vi "List_Files.vi"(8 "error in (no error)":errorcluster, 11 "IB_Source_File in":refnum<class "IB_Source_File.lvclass">) -> (0 "error out":errorcluster, 3 "Files":T1[](array[typedef]))   [LabVIEW 2020, in "IB_Source_File.lvclass"]
uses:
  <vilib>/AppBuilder/IB_Classes/Source/File/IB_Source_File.lvclass
  <vilib>/AppBuilder/IB_Classes/Source/File/IB_Source_File.lvclass/IB_Source_File.ctl
  <resource>/Framework/Providers/Builds/Installer/CDK_sTypeDef_FileList.ctl
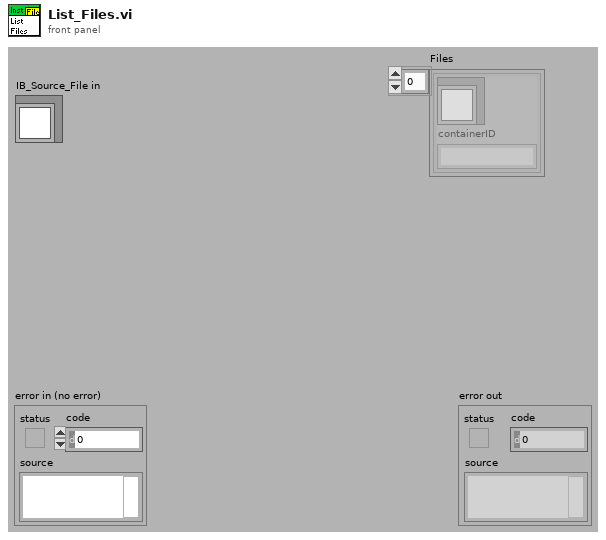
[diagram p1: front panel]
types:
  T1 = typedef "CDK_sTypeDef_FileList.ctl" = cluster{"FileInventory":refnum<class "IB_Source_File.lvclass">, "containerID":string}
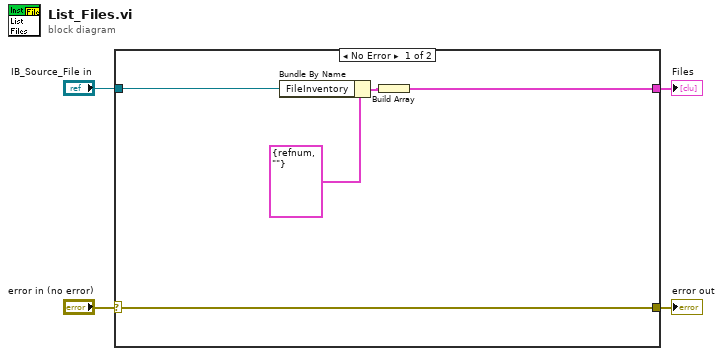
[diagram p0: block diagram]
diagram:
  n1 = case shown="No Error" "error in (no error)" {
    selector: "error in (no error)" -> [w9 w10]
    tunnel: [w9 w10] -> w3
    tunnel: "IB_Source_File in" -> [w6 _]
    tunnel: [w8 _] -> w1
    frame No Error {
      n2 = Bundle By Name(cluster=T1 {"FileInventory"=refnum, "containerID"=""} ("files"), "FileInventory"=w6) -> (w5:T1)
      n3 = Build Array(w5) -> (w8:T1[])
    }
    frame Error {
    }
  }
  "error out" <- w3
  "Files" <- w1
